vi "write boolean and numeric Vaues .vi"() -> ()   [LabVIEW 2016]
panel:
  in  "Numeric":dbl
  in  "M0":bool
  in  "stop":bool
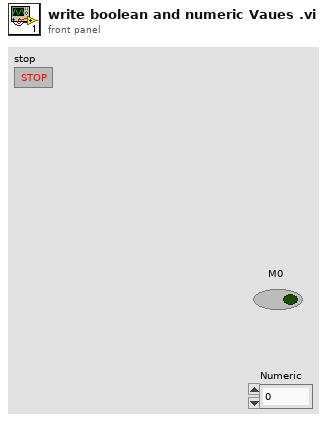
[diagram p1: front panel]
types:
  T1 = enum16{"Read", "Write", "ReadWrite", "BufferedRead", "BufferedReadWrite"}
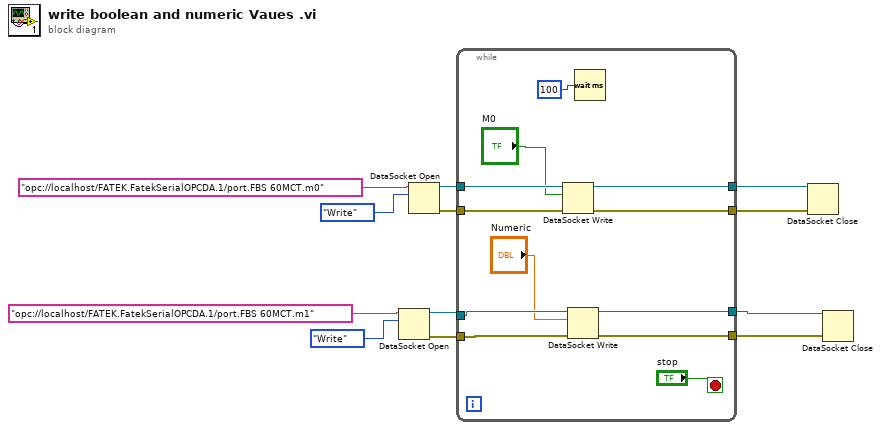
[diagram p0: block diagram]
diagram:
  n1 = DataSocket Open(10:T1."Write" ("mode"), 11:"opc://localhost/FATEK.FatekSerialOPCDA.1/port.FBS 60MCT.m1") -> (0:w3:errorcluster, 3:w4:refnum<k13>)  [unwired: 2 in]
  n2 = DataSocket Open(10:T1."Write" ("mode"), 11:"opc://localhost/FATEK.FatekSerialOPCDA.1/port.FBS 60MCT.m0") -> (0:w11:errorcluster, 3:w10:refnum<k13>)  [unwired: 2 in]
  n3 = while {
    tunnel: w11 -> [w23]
    tunnel: w10 -> [w22]
    tunnel: [w21] -> w9
    tunnel: [w20] -> w8
    tunnel: w4 -> [w17]
    tunnel: w3 -> [w16]
    tunnel: [w15] -> w2
    tunnel: [w14] -> w1
    stop <- "stop" stop-if-true
    n4 = DataSocket Write(8:w23, 10:"M0", 11:w22) -> (0:w21:errorcluster, 3:w20:refnum<k13>)  [unwired: 1 in, 1 out]
    n5 = DataSocket Write(8:w16, 10:"Numeric", 11:w17) -> (0:w14:errorcluster, 3:w15:refnum<k13>)  [unwired: 1 in, 1 out]
    n6 = Wait (ms)(milliseconds to wait=u32 100) -> ()  [unwired: 1 out]
  }
  n7 = DataSocket Close(8:w9, 11:w8) -> ()  [unwired: 1 in, 2 out]
  n8 = DataSocket Close(8:w1, 11:w2) -> ()  [unwired: 1 in, 2 out]
